vi "lua_rawlen.vi"(8 "error in (no error)":errorcluster, 10 "index":i32, 11 "lua_state_p":u64) -> (0 "error out":errorcluster, 2 "length":u64, 3 "lua_state_p out":u64)   [LabVIEW 2020, in "lua.dll.lvlib"]
doc: "Returns the raw \"length\" of the value at the given index: for strings, this is the string length; for tables, this is the result of the length operator ('#') with no metamethods; for userdata, this is the size of the block of memory allocated for the userdata; for other values, it is 0."
uses:
  lua.dll.lvlib
  lua54.dll
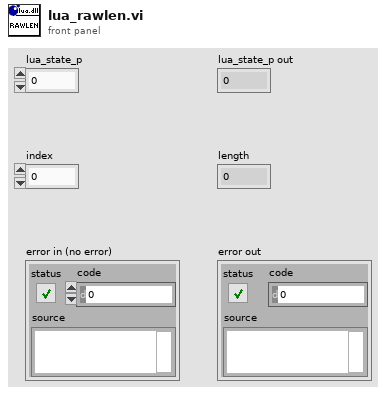
[diagram p1: front panel]
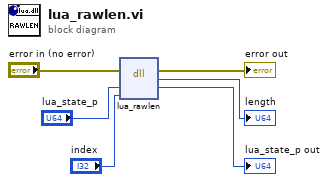
[diagram p0: block diagram]
diagram:
  n1 = dll-call lib="C:/Users/Nicholas Folse/Documents/workspace/github-tauterra.llc/Lua for LabVIEW/lib/lua.dll/lua54**.*" fn="lua_rawlen"(error in="error in (no error)", "lua_state_p"="lua_state_p", "index"="index") -> (error out=→"error out":errorcluster, "rawlen"=→"length":u64, "lua_state_p"=→"lua_state_p out":u64)  [unwired: 3 in, 1 out]
